vi "Write Scheduled Tx Channel.vi"(6 "data in":u32[](array[numeric]), 8 "error in":errorcluster, 9 "labels settings for RT":T1[](array[typedef]) {"Label Timestamp Channel Data Reference" format="%.0x"; "Word Initial Raw Value" format="%032.0f"; "Label Disable/Trigger Channel Reference" format="%.0x"; "parameter driver data"."Tx parameter refs" format="%.0x"; "SDI" format="%02b"; "label" format="%.0o"}, 10 "channel number in":u8, 11 "board handle in":u8) -> (0 "error out":errorcluster, 2 "channel number out":u8, 3 "board handle out":u8)   [LabVIEW 2020, in "AIM ARINC 429 Hardware API.lvlib"]
uses:
  AIM ARINC 429 Hardware API.lvlib
  <instrlib>/AIM GmbH/_ARINC-429/AIM429LV.lvlib
  Shared/Label.ctl
  <vilib>/NI/NI VeriStand Encoding and Decoding/Encoding.ctl
  <vilib>/NI/NI VeriStand Encoding and Decoding/Encoding and Decoding.lvlib
  Shared/Parameter Definition.ctl
  <vilib>/NI VeriStand/Custom Device API/Custom Device Item Ref.ctl
  <vilib>/NI VeriStand/Custom Device API/Custom Device API.lvlib
  Shared/RT Parameters.ctl
  Shared/Transfer Type.ctl
  <vilib>/NI VeriStand/Custom Device API/Data Reference.ctl
  Shared/RT Label Settings.ctl
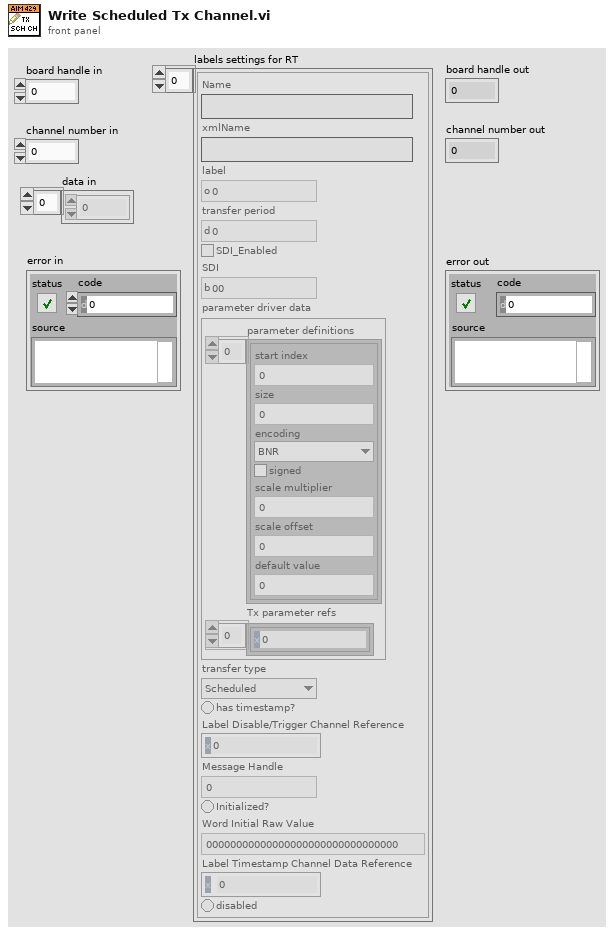
[diagram p1: front panel]
types:
  T1 = typedef "RT Label Settings.ctl" = cluster{"Name":string, "xmlName":string, "label":T2, "transfer period":u32, "SDI_Enabled":bool, "SDI":u8, "parameter driver data":T3, "transfer type":T7, "has timestamp?":bool, "Label Disable/Trigger Channel Reference":T6, "Message Handle":u64, "Initialized?":bool, "Word Initial Raw Value":u32, "Label Timestamp Channel Data Reference":T8, "disabled":bool}
  T2 = typedef "Label.ctl" = u8
  T3 = typedef "RT Parameters.ctl" = cluster{"parameter definitions":T4[], "Tx parameter refs":T6[]}
  T4 = typedef "Parameter Definition.ctl" = cluster{"start index":i32, "size":i32, "encoding":T5, "signed":bool, "scale multiplier":dbl, "scale offset":dbl, "default value":dbl}
  T5 = typedef "Encoding and Decoding.lvlib/Encoding.ctl" = enum16{"BNR", "BCD", "Discrete"}
  T6 = typedef "Custom Device API.lvlib/Custom Device Item Ref.ctl" = u64
  T7 = typedef "Transfer Type.ctl" = enum16{"Scheduled", "Acyclic", "Block", "Strobe"}
  T8 = typedef "Custom Device API.lvlib/Data Reference.ctl" = i32
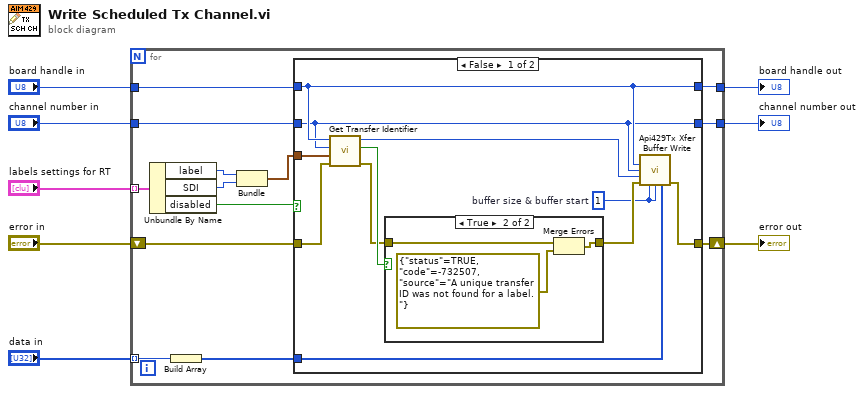
[diagram p0: block diagram]
diagram:
  n1 = for {
    tunnel: "board handle in" -> [w15]
    tunnel: "channel number in" -> [w16]
    tunnel: "labels settings for RT" -> [w21] mode=indexing
    shift-right: [w17] -> w3
    shift-left: "error in" -> [w20]
    tunnel: "data in" -> [w19] mode=indexing
    tunnel: [w12] -> w2
    tunnel: [w13] -> w1
    n2 = Unbundle By Name(w21) -> ("label"=w11:T2, "SDI"=w10:u8, "disabled"=w14:bool)
    n3 = Build Array(w19) -> (w18:u32[])
    n4 = Bundle("label"=w11, "SDI"=w10) -> (w9:cluster{"label":T2, "SDI":u8})  [unwired: 1 in]
    n5 = case shown="False" w14 {
      tunnel: w9 -> [w32 _]
      tunnel: w20 -> [w31 w39]
      tunnel: w18 -> [w25 _]
      tunnel: [w24 w39] -> w17
      tunnel: w16 -> [w22 w37]
      tunnel: w15 -> [w23 w38]
      tunnel: [w23 w38] -> w13
      tunnel: [w22 w37] -> w12
      frame False {
        w26 = u16 1  # buffer size & buffer start
        n6 = call "Get Transfer Identifier.vi"("error in"=w31, "label information"=w32, "channel number in"=w22, "board number in"=w23) -> ("error out"=w29:errorcluster, "new entry created"=w30:bool, "Transfer ID out"=w28:u32)  [unwired: 5 in]
        n7 = case shown="True" w30 {
          tunnel: w29 -> [w33 w36]
          tunnel: [w33 w34] -> w27
          frame False {
          }
          frame True {
            n8 = Merge Errors(w36, errorcluster {"status"=TRUE, "code"=-732507, "source"="A unique transfer ID was not found for a label."} ("error constant")) -> (w34:errorcluster)
          }
        }
        n9 = call <instrlib>:"Api429Tx Xfer Buffer Write.vi"("board_handle"=w23, "b_Chn"=w22, "ul_XferId"=w28, "error in (no error)"=w27, "w_BufStart"=w26, "w_BufSize"=w26, "pl_LData"=w25) -> ("error out"=w24:errorcluster)  [unwired: 8 in]
      }
      frame True {
        # "do not write data if label is disabled"
      }
    }
  }
  "board handle out" <- w1
  "channel number out" <- w2
  "error out" <- w3
